vi "Shutdown Control Loop.vi"   [LabVIEW 2014]
uses:
  <vilib>/Platform/TimedLoop/XDataNode/timing_clust.ctl
  <vilib>/Platform/TimedLoop/XDataNode/nitl_modes.ctl
  <vilib>/Platform/TimedLoop/XDataNode/wakeup.ctl
  Vehicle Status/Subsystem Status.ctl
  Reason for Shutdown.ctl
  <vilib>/FPGAPlugInAG/sbRIO-9626/niLvFpga_Open_sbRIO-9626.vi
  Global Data.vi
  <vilib>/Utility/error.llb/Error Cluster From Error Code.vi
  <vilib>/rvi/errors/niLvFpgaAdjustHostInterfaceError.vi
  <vilib>/rvi/interface/nirviOpenFPGA/nirviOpenFPGA.xnode
  FPGA Bitfiles/FormulaElectric2_FPGATarget_FPGA_8a5J0mMac2U.lvbitx
  <vilib>/Platform/TimedLoop/XDataNode/XDataNode.xnode
  <vilib>/rvi/interface/nirviReadWriteControl/nirviReadWriteControl.xnode
  FPGA Typedef.ctl
  Dash LED Status.ctl
  <vilib>/Platform/TimedLoop/XDataNode/XDNodeRunTimeDep.lvlib
  NiFpgaLv.dll
types:
  T1 = typedef "XDNodeRunTimeDep.lvlib/timing_clust.ctl" = cluster{"Expected End [f-1]":u64, "Actual End [f-1]":u64, "Finished Late? [f-1]":bool, "Expected End [i-1]":u64, "Actual End [i-1]":u64, "Finished Late? [i-1]":bool, "Expected Start [i]":u64, "Actual Start [i]":u64, "Expected Start [f]":u64, "Actual Start [f]":u64, "Source Name":string, "Structure Name":string, "Period":i64, "Deadline":i64, "Offset":i64, "Start":i64, "Priority":i32, "Timeout":i32, "Mode":T2, "Wakeup Reason":T3, "Error":errorcluster, "Source Type":string, "Secondary Source Type":string, "Global End Time":u64, "Global Start Time":u64, "Frame Duration":u64, "Iteration Duration":u64, "Assigned CPU":i32, "I/O Scan Engine Mode":u32}
  T2 = typedef "XDNodeRunTimeDep.lvlib/nitl_modes.ctl" = enum32{"No Change", "Process missed periods, maintain original phase", "Discard missed periods, maintain original phase", "Process missed periods, ignore original phase", "Discard missed periods, ignore original phase"}
  T3 = typedef "XDNodeRunTimeDep.lvlib/wakeup.ctl" = enum32{"Normal", "Aborted", "Asynchronous wakeup", "Timing source error", "Timed loop error", "Timeout"}
  T4 = typedef "Subsystem Status.ctl" = enum16{"Okay", "Short Warning", "Long Warning", "Return to Pits", "Error", "Danger"}
  T5 = typedef "Reason for Shutdown.ctl" = enum16{"None", "BMS", "Shutdown", "sbRIO", "MC", "Remote"}
  T6 = typedef "FPGA Typedef.ctl" = refnum<k20>
  T7 = typedef "Dash LED Status.ctl" = enum16{"Off", "Flashing", "On"}
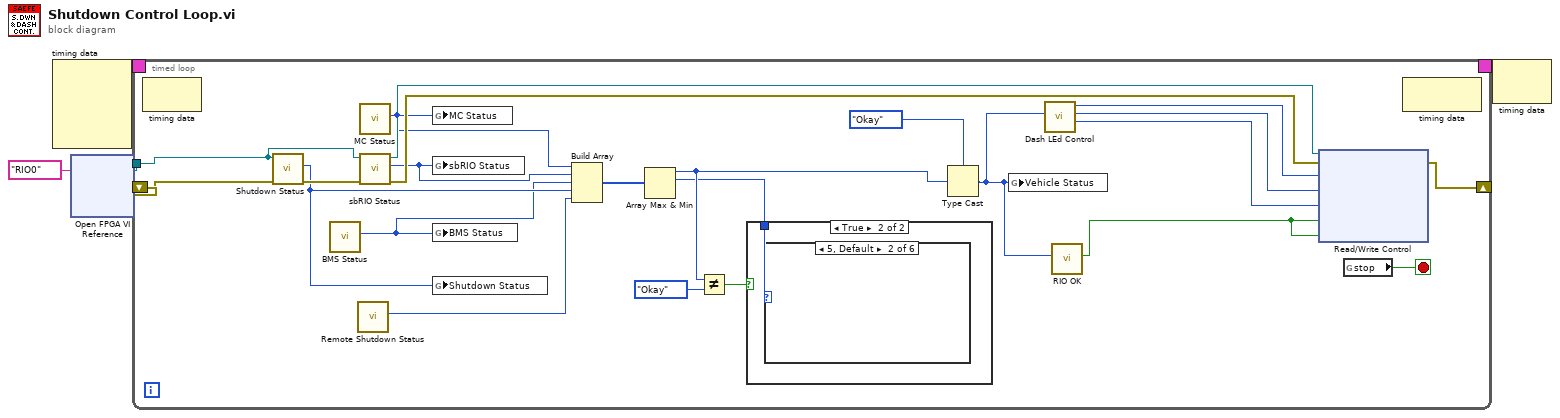
[diagram p0: block diagram]
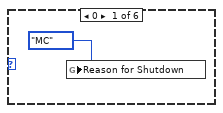
[diagram p3: hidden frame]
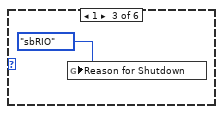
[diagram p4: hidden frame]
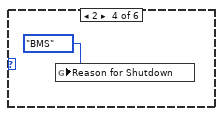
[diagram p5: hidden frame]
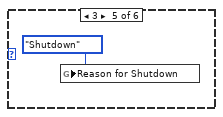
[diagram p6: hidden frame]
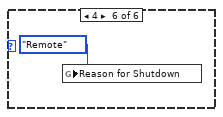
[diagram p7: hidden frame]
diagram:
  n1 = node-c288() -> (w4:T1)  [unwired: 4 in]
  n2 = xnode "Open FPGA VI Reference"("resource name"=tag "RIO0") -> ("FPGA VI Reference Out"=w2:refnum<k20>, "error out"=w5:errorcluster)  [unwired: 1 in]
  n3 = timed-loop {
    shift-right: [w21] -> _
    shift-left: w5 -> [w28]
    timing: w4 -> [_]
    timing-out: [_] -> w3
    tunnel: w2 -> [w18]
    stop <- w20 stop-if-true
    n4 = node-c288() -> ()  [unwired: 1 in, 1 out]
    n5 = call "Shutdown Status.vi"("error in"=w28, "FPGA VI Reference In"=w18) -> ("error out"=w27:errorcluster, "Subsystem Status"=w13:T4)  [unwired: 7 in, 1 out]
    n6 = call "BMS Status.vi"() -> ("Subsystem Status"=w6:T4)  [unwired: 11 in]
    n7 = call "Remote Shutdown Status.vi"() -> ("Subsystem Status"=w12:T4)  [unwired: 11 in]
    n8 = call "MC Status.vi"() -> ("Subsystem Status"=w15:T4)  [unwired: 11 in]
    n9 = call "sbRIO Status.vi"("error in (no error)"=w27, "Refnum in"=w18) -> ("error out"=w25:errorcluster, "Subsystem Status"=w14:T4, "Refnum out"=w19:T6)  [unwired: 7 in]
    n10 = global write "Global Data.vi" "MC Status"(w15) -> ()
    n11 = global write "Global Data.vi" "sbRIO Status"(w14) -> ()
    n12 = global write "Global Data.vi" "BMS Status"(w6) -> ()
    n13 = global write "Global Data.vi" "Shutdown Status"(w13) -> ()
    n14 = Build Array(w15, w14, w6, w13, w12) -> (w11:T4[])
    n15 = Array Max & Min(array=w11) -> (max value=w9:T4, max index (indices)=w7:i32)  [unwired: 2 out]
    n16 = Not Equal?(x=w9, y=Subsystem_Status."Okay") -> (x != y?=w10:bool)
    n17 = case shown="True" w10 {
      tunnel: w7 -> [_ w29]
      frame False {
      }
      frame True {
        n18 = case shown="5, Default" w29 {
          frame 0 {
            n19 = global write "Global Data.vi" "Reason for Shutdown"(Reason_for_Shutdown."MC" ("Reason for Shutdown")) -> ()
          }
          frame 5, Default {
          }
          frame 1 {
            n20 = global write "Global Data.vi" "Reason for Shutdown"(Reason_for_Shutdown."sbRIO" ("Reason for Shutdown")) -> ()
          }
          frame 2 {
            n21 = global write "Global Data.vi" "Reason for Shutdown"(Reason_for_Shutdown."BMS" ("Reason for Shutdown")) -> ()
          }
          frame 3 {
            n22 = global write "Global Data.vi" "Reason for Shutdown"(Reason_for_Shutdown."Shutdown" ("Reason for Shutdown")) -> ()
          }
          frame 4 {
            n23 = global write "Global Data.vi" "Reason for Shutdown"(Reason_for_Shutdown."Remote" ("Reason for Shutdown")) -> ()
          }
        }
      }
    }
    n24 = Type Cast(type=Subsystem_Status."Okay" ("Subsystem Status"), x=w9) -> (*(type *) &x=w17:T4)
    n25 = global write "Global Data.vi" "Vehicle Status"(w17) -> ()
    n26 = call "Dash LEd Control.vi"("Vehicle Status"=w17) -> ("Red LED"=w22:T7, "Yellow LED"=w23:T7, "Green LED"=w24:T7)  [unwired: 8 in]
    n27 = call "RIO OK.vi"("Vehicle Status"=w17) -> ("RIO OK"=w16:bool)  [unwired: 10 in]
    n28 = xnode "Read/Write Control"("FPGA VI Reference In"=w19, "error in"=w25, "Green LED"=w24, "Yellow LED"=w23, "Red LED"=w22, "cRIO Shutdown 1"=w16, "cRIO Shutdown 2"=w16) -> ("error out"=w21:errorcluster)  [unwired: 1 out]
    n29 = global read "Global Data.vi" "stop"() -> (w20:bool)
    n30 = node-c288() -> ()  [unwired: 1 in, 1 out]
  }
  n31 = node-c288(w3) -> ()  [unwired: 1 out]
